vi "VCOControl.vi"() -> ()   [LabVIEW 2014]
uses:
  <vilib>/DAQmx/create/channels.llb/DAQmx Create Channel (AI-Voltage-Basic).vi
  <vilib>/DAQmx/configure/timing.llb/DAQmx Timing (Sample Clock).vi
  <vilib>/DAQmx/create/channels.llb/DAQmx Create Channel (AO-Voltage-Basic).vi
  <vilib>/DAQmx/write.llb/DAQmx Write (Analog DBL 1Chan 1Samp).vi
  <vilib>/DAQmx/read.llb/DAQmx Read (Analog Wfm 1Chan NSamp).vi
  <vilib>/measure/matone.llb/Extract Single Tone Information 1 Chan.vi
  <vilib>/addons/control/pid/pid.llb/PID (DBL).vi
  <vilib>/measure/NI_MAPro.lvlib
  <vilib>/addons/control/pid/NI_PID_pid.lvlib
panel:
  in  "PID gains":T1={"proportional gain (Kc)"=1.0, "integral time (Ti, min)"=0.01, "derivative time (Td, min)"=0.0} {"derivative time (Td, min)" format="%.3f"; "integral time (Ti, min)" format="%.3f"; "proportional gain (Kc)" format="%.3f"}
  in  "Setpoint Frequency":dbl format="%.2f"
  in  "stop":bool
  in  "AO Channel":tag
  in  "AI Channel":tag
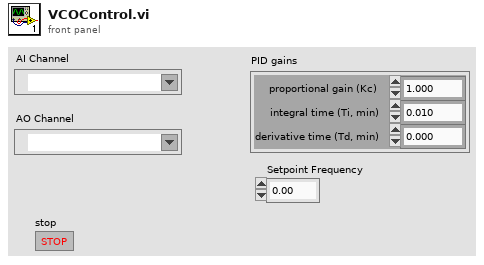
[diagram p1: front panel]
types:
  T1 = cluster{"proportional gain (Kc)":dbl, "integral time (Ti, min)":dbl, "derivative time (Td, min)":dbl}
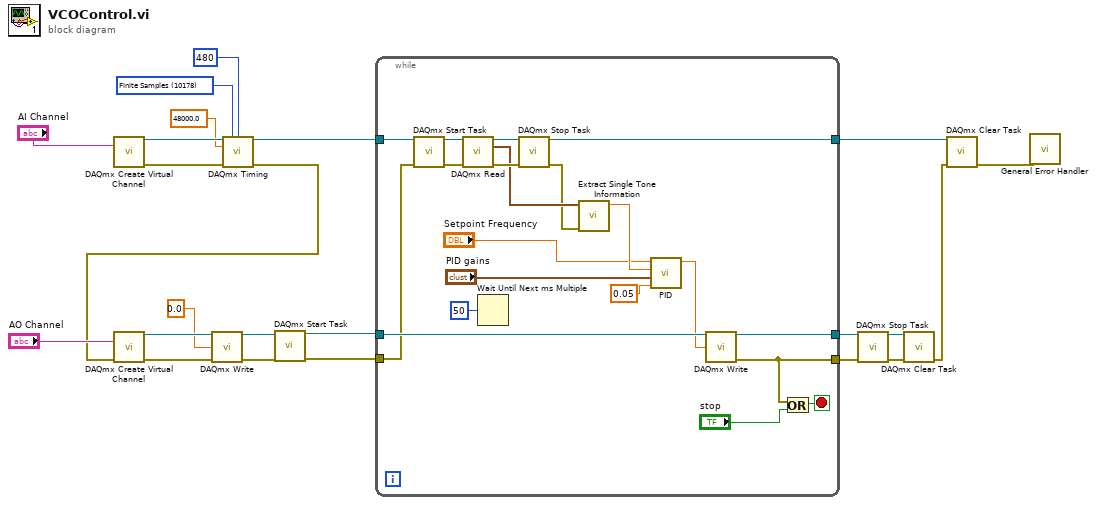
[diagram p0: block diagram]
diagram:
  w20 = 10178 items=["Finite Samples"=10178, "Continuous Samples"=10123, "Hardware Timed Single Point"=12522] ("sample mode")
  n1 = call-poly <vilib>:"DAQmx Create Virtual Channel.vi"("physical channels"="AI Channel") -> ("task out"=w22:refnum<k21>, "error out"=w21:errorcluster)  [unwired: 13 in]
  n2 = call-poly <vilib>:"DAQmx Timing.vi"("task/channels in"=w22, "sample mode"=w20, "samples per channel"=480, "rate"=48000.0, "error in"=w21) -> ("task out"=w17:refnum<k21>, "error out"=w2:errorcluster)  [unwired: 9 in]
  n3 = call-poly <vilib>:"DAQmx Create Virtual Channel.vi"("physical channels"="AO Channel", "error in"=w2) -> ("task out"=w7:refnum<k21>, "error out"=w5:errorcluster)  [unwired: 12 in]
  n4 = call-poly <vilib>:"DAQmx Write.vi"("task/channels in"=w7, "data"=0.0, "error in"=w5) -> ("task out"=w6:refnum<k21>, "error out"=w4:errorcluster)  [unwired: 10 in, 1 out]
  n5 = call <vilib>:"DAQmx Start Task.vi"("task/channels in"=w6, "error in"=w4) -> ("task out"=w13:refnum<k21>, "error out"=w12:errorcluster)  [unwired: 12 in]
  n6 = while {
    tunnel: w17 -> [w43]
    tunnel: [w38] -> w16
    tunnel: w13 -> [w37]
    tunnel: w12 -> [w35]
    tunnel: [w36] -> w11
    tunnel: [w33] -> w10
    stop <- w34 stop-if-true
    n7 = call <vilib>:"DAQmx Start Task.vi"("task/channels in"=w43, "error in"=w35) -> ("task out"=w42:refnum<k21>, "error out"=w41:errorcluster)  [unwired: 12 in]
    n8 = call-poly <vilib>:"DAQmx Read.vi"("task/channels in"=w42, "error in"=w41) -> ("task out"=w40:refnum<k21>, "data"=w31:waveform(dbl), "error out"=w39:errorcluster)  [unwired: 11 in]
    n9 = Wait Until Next ms Multiple(millisecond multiple=u32 50) -> ()  [unwired: 1 out]
    n10 = call <vilib>:"DAQmx Stop Task.vi"("task/channels in"=w40, "error in"=w39) -> ("task out"=w38:refnum<k21>, "error out"=w30:errorcluster)  [unwired: 12 in]
    n11 = call-poly <vilib>:"Extract Single Tone Information.vi"("error in (no error)"=w30, "time signal in"=w31) -> ("detected frequency"=w29:dbl)  [unwired: 4 in, 5 out]
    n12 = call-poly <vilib>:"PID.vi"("dt (s)"=0.05, "PID gains"="PID gains", "process variable"=w29, "setpoint"="Setpoint Frequency") -> ("output"=w26:dbl)  [unwired: 6 in, 1 out]
    n13 = call-poly <vilib>:"DAQmx Write.vi"("task/channels in"=w37, "data"=w26) -> ("task out"=w36:refnum<k21>, "error out"=w33:errorcluster)  [unwired: 11 in, 1 out]
    n14 = Or(x=w33, y="stop") -> (x .or. y?=w34:bool)
  }
  n15 = call <vilib>:"DAQmx Stop Task.vi"("task/channels in"=w11, "error in"=w10) -> ("task out"=w9:refnum<k21>, "error out"=w8:errorcluster)  [unwired: 12 in]
  n16 = call <vilib>:"DAQmx Clear Task.vi"("task in"=w9, "error in"=w8) -> ("error out"=w1:errorcluster)  [unwired: 13 in]
  n17 = call <vilib>:"DAQmx Clear Task.vi"("task in"=w16, "error in"=w1) -> ("error out"=w15:errorcluster)  [unwired: 13 in]
  n18 = call <vilib>:"General Error Handler.vi"("error in (no error)"=w15) -> ()  [unwired: 10 in, 5 out]
